vi "Symmetrize (multiple).vi"(8 "error in (no error)":errorcluster, 11 "XY-data":cluster{"X-array":dbl[], "Y-array":dbl[]}[](array[cluster]) {"Y-array" format="%.2p"; "X-array" format="%.2p"}) -> (0 "error out":errorcluster, 1 "Antisymmetric":cluster{"X-array":dbl[], dbl[]}[](array[cluster]), 2 "Symmetric":cluster{"X-array":dbl[], dbl[]}[](array[cluster]), 3 "XY-data out":cluster{"X-array":dbl[], "Y-array":dbl[]}[](array[cluster]) {"Y-array" format="%.2p"; "X-array" format="%.2p"})   [LabVIEW 2019, in "xy_utilities.lvlib"]
doc: "Compute the Symmetric and Antisymmetric functions of <b>XY-data</b>\n\n<b>Symmetric</b>: f+ = (f(x) + f(-x))/2\n<b>Antisymmetric</b>: f- = (f(x) - f(-x))/2"
uses:
  xy_utilities.lvlib
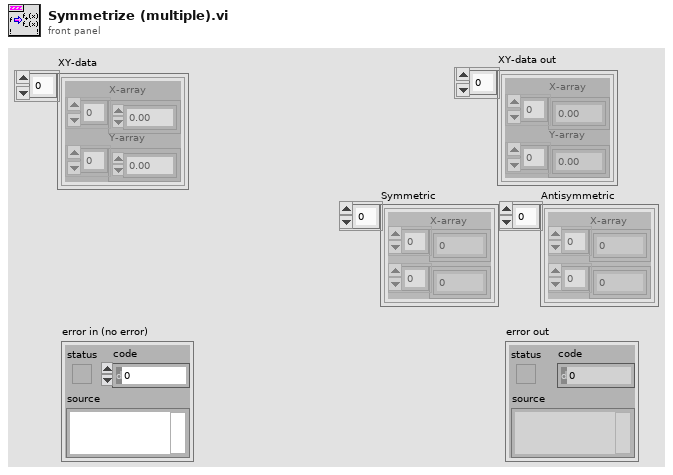
[diagram p1: front panel]
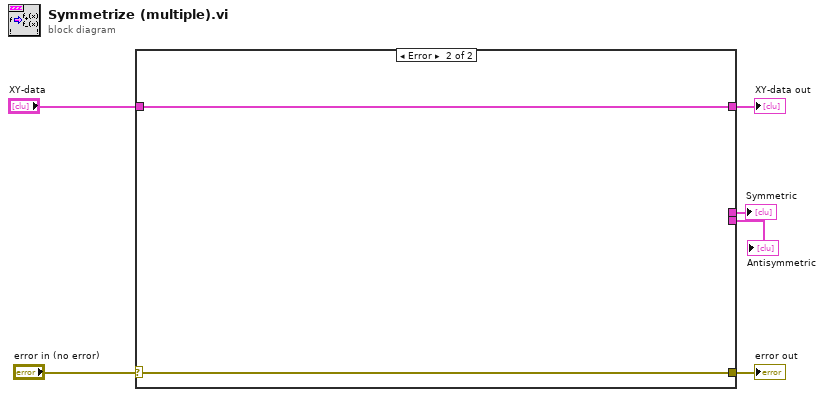
[diagram p0: block diagram]
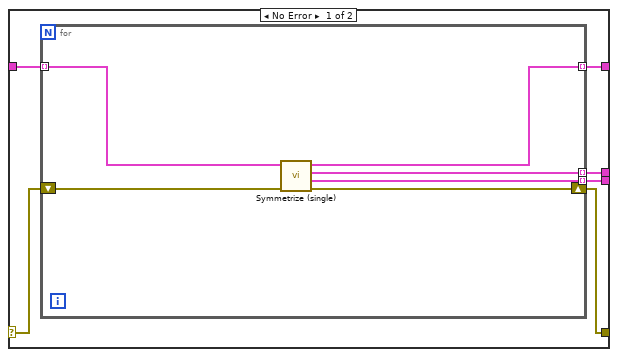
[diagram p2: hidden frame]
diagram:
  n1 = case shown="Error" "error in (no error)" {
    selector: "error in (no error)" -> [w8 w20]
    tunnel: [w7 w20] -> w5
    tunnel: "XY-data" -> [w12 w19]
    tunnel: [w11 w19] -> w3
    tunnel: [w10 _] -> w2
    tunnel: [w9 _] -> w1
    frame No Error {
      n2 = for {
        tunnel: w12 -> [w18] mode=indexing
        tunnel: [w17] -> w11 mode=indexing
        tunnel: [w16] -> w10 mode=indexing
        tunnel: [w15] -> w9 mode=indexing
        shift-right: [w14] -> w7
        shift-left: w8 -> [w13]
        n3 = call "Symmetrize (single).vi"("error in (no error)"=w13, "XY-data"=w18) -> ("error out"=w14:errorcluster, "Antisymmetric"=w15:cluster{"X-array":dbl[], dbl[]}, "Symmetric"=w16:cluster{"X-array":dbl[], dbl[]}, "XY-data out"=w17:cluster{"X-array":dbl[], "Y-array":dbl[]})  [unwired: 6 in]
      }
    }
    frame Error {
    }
  }
  "error out" <- w5
  "XY-data out" <- w3
  "Symmetric" <- w2
  "Antisymmetric" <- w1
